vi "TIO Stream Close.vi"(8 "error in (no error)":errorcluster, 11 "TS Connection":T1={"Type"=enum."TCP", "Serial"="serial:///dev/cu.usbserial-00000", "TCP"=refnum, "Timeout"=500}) -> ()   [LabVIEW 2016]
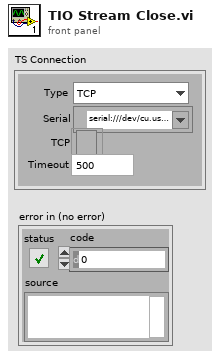
[diagram p1: front panel]
types:
  T1 = cluster{"Type":enum16{"TCP", "Serial"}, "Serial":refnum<visa-resource-name>, "TCP":refnum<k5>, "Timeout":u32}
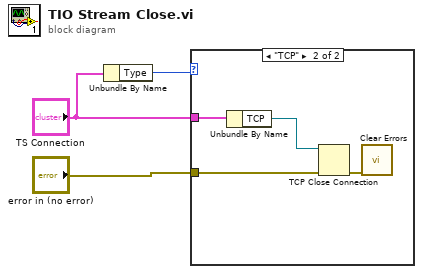
[diagram p0: block diagram]
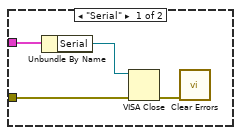
[diagram p2: hidden frame]
diagram:
  n1 = Unbundle By Name("TS Connection") -> ("Type"=w2:enum16{"TCP", "Serial"})
  n2 = case shown="\"TCP\"" w2 {
    tunnel: "error in (no error)" -> [w7 w10]
    tunnel: "TS Connection" -> [w5 w11]
    frame "Serial" {
      n3 = Unbundle By Name(w5) -> ("Serial"=w4:refnum<visa-resource-name>)
      n4 = VISA Close(VISA resource name=w4, error in (no error)=w7) -> (error out=w6:errorcluster)
      n5 = call <vilib>:"Clear Errors.vi"("error in (no error)"=w6) -> ()  [unwired: 5 in, 2 out]
    }
    frame "TCP" {
      n6 = Unbundle By Name(w11) -> ("TCP"=w8:refnum<k5>)
      n7 = TCP Close Connection(connection ID=w8, error in (no error)=w10) -> (error out=w9:errorcluster)  [unwired: 1 in, 1 out]
      n8 = call <vilib>:"Clear Errors.vi"("error in (no error)"=w9) -> ()  [unwired: 5 in, 2 out]
    }
  }
